vi "Template.vi"() -> ()   [LabVIEW 2021]
uses:
  _Template/_Template/_Template.lvclass
  _Shared/_Shared.lvlib
panel:
  in  "Create":bool
  in  "Template Name":string(combo)
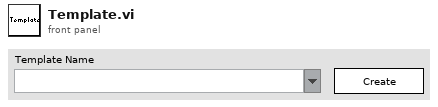
[diagram p1: front panel]
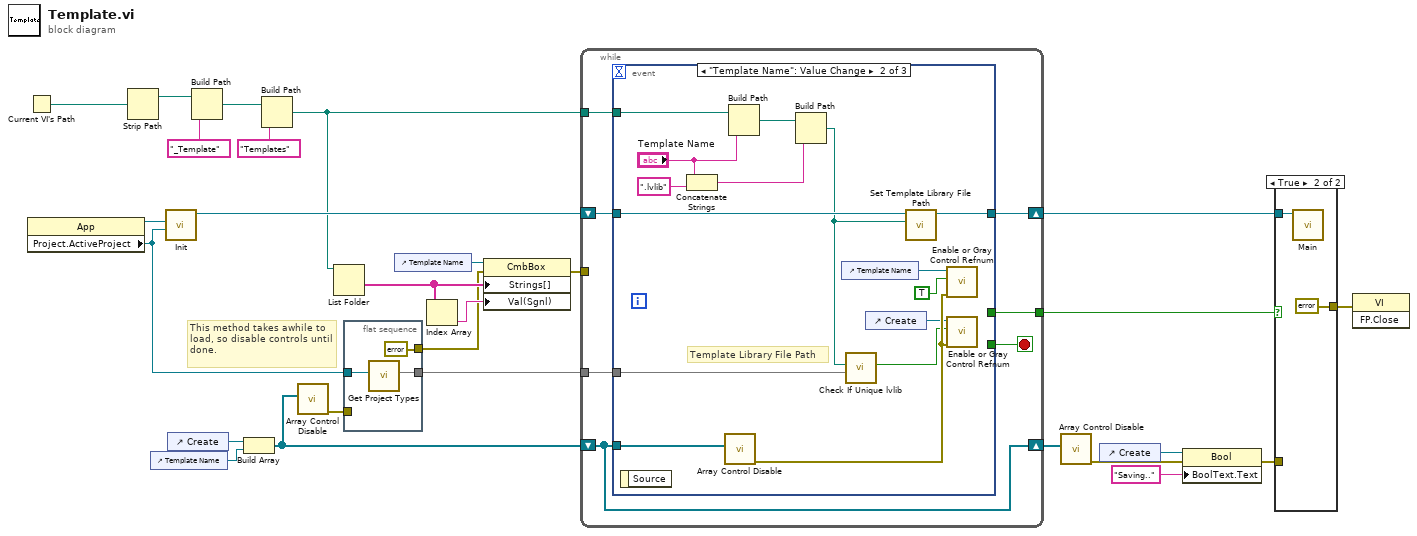
[diagram p0: block diagram]
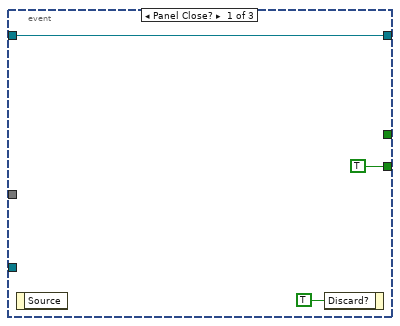
[diagram p2: hidden frame]
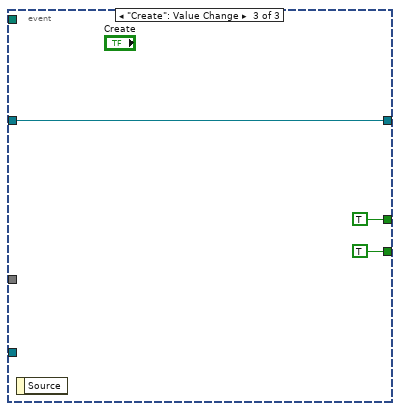
[diagram p3: hidden frame]
diagram:
  # "This method takes awhile to load, so disable controls until done."
  n1 = Current VI's Path() -> (path=w25:path)
  n2 = property class="App"() -> (reference out=w17:refnum<vi>, "Project.ActiveProject"=w14:refnum<vi>)  [unwired: 2 in, 1 out]
  n3 = Strip Path(path=w25) -> (stripped path=w21:path)  [unwired: 1 out]
  n4 = control-ref of="Template Name"() -> (w6:refnum<vi>)
  n5 = call "Init.vi"("Project:Active Project"=w14, "NI.LV.Dialog Instance"=w17) -> ("_Template out"=w18:refnum<class "_Template.lvclass">)  [unwired: 9 in]
  n6 = control-ref of="Create"() -> (w7:refnum<vi>)
  n7 = Build Path(base path=w21, name or relative path="_Template" ("regular expression")) -> (appended path=w22:path)
  n8 = Build Array(w7, w6) -> (w5:refnum<vi>[])
  n9 = Build Path(base path=w22, name or relative path="Templates" ("regular expression")) -> (appended path=w15:path)
  n10 = call "Array Control Disable.vi"("Array Control in"=w5) -> ("error out"=w4:errorcluster)  [unwired: 10 in]
  n11 = List Folder(path=w15) -> (folder names=w11:string[])  [unwired: 3 in, 3 out]
  n12 = flat-sequence {
    tunnel: w14 -> [w30]
    tunnel: [w29] -> w13
    tunnel: [errorcluster {"status"=FALSE, "code"=0, "source"=""} ("error out")] -> w10
    tunnel: w4 -> [_]
    frame #0 {
      n13 = call "Get Project Types.vi"("Project:Active Project"=w30) -> ("Type Name Library File Path"=w29:map{string, map{string, path}})  [unwired: 10 in]
    }
  }
  n14 = control-ref of="Template Name"() -> (w26:refnum<vi>)
  n15 = Index Array(array=w11) -> (element=w12:string)  [unwired: 1 in]
  n16 = property class="CmbBox"(reference=w26, error in=w10, "Strings[]"=w11, "Val(Sgnl)"=w12) -> (error out=w19:errorcluster)  [unwired: 1 out]
  n17 = while {
    tunnel: [w37] -> w27
    tunnel: w19 -> [_]
    shift-right: [w34] -> w16
    shift-left: w18 -> [w35]
    tunnel: w15 -> [w33]
    tunnel: w13 -> [w32]
    shift-right: [w31] -> w3
    shift-left: w5 -> [w31]
    stop <- w36 stop-if-true
    n18 = event shown="[1] \"Template Name\": Value Change" {
      selector: _ -> [_ _ _]
      dyn-events: _ -> [_ _ _]
      timeout: _ -> [_ _ _]
      tunnel: [_ _ TRUE] -> w37
      tunnel: [TRUE ("Discard?") _ TRUE ("Discard?")] -> w36
      tunnel: w35 -> [w38 w48 w56]
      tunnel: [w38 w47 w56] -> w34
      tunnel: w33 -> [_ w53 _]
      tunnel: w32 -> [_ w46 _]
      tunnel: w31 -> [_ w42 _]
      event Panel Close? {
        n19 = event-data() -> ()  [unwired: 1 in, 1 out]
        n20 = event-data("Discard?"=TRUE) -> ()  [unwired: 1 in, 1 out]
      }
      event "Template Name": Value Change {
        # "Template Library File Path"
        n21 = event-data() -> ()  [unwired: 1 in, 1 out]
        n22 = Concatenate Strings("Template Name", ".lvlib" ("string")) -> (w51:string)
        n23 = call "Array Control Disable.vi"("Array Control in"=w42) -> ("error out"=w55:errorcluster)  [unwired: 10 in]
        n24 = Build Path(base path=w53, name or relative path="Template Name") -> (appended path=w52:path)
        n25 = Build Path(base path=w52, name or relative path=w51) -> (appended path=w45:path)
        n26 = control-ref of="Template Name"() -> (w43:refnum<vi>)
        n27 = call "Check If Unique lvlib.vi"("Type Name Library File Path"=w46, "Library File Path"=w45) -> ("Unique?"=w41:bool)  [unwired: 9 in]
        n28 = control-ref of="Create"() -> (w49:refnum<vi>)
        n29 = call "Set Template Library File Path.vi"("Template Library File Path"=w45, "_Template in"=w48) -> ("_Template out"=w47:refnum<class "_Template.lvclass">)  [unwired: 9 in]
        n30 = call <vilib>:"Enable or Gray Control Refnum.vi"("error in (no error)"=w55, "enable?"=TRUE, "Control in"=w43) -> ()  [unwired: 7 in, 2 out]
        n31 = call <vilib>:"Enable or Gray Control Refnum.vi"("error in (no error)"=w55, "enable?"=w41, "Control in"=w49) -> ()  [unwired: 7 in, 2 out]
      }
      event "Create": Value Change {
        n32 = event-data() -> ()  [unwired: 1 in, 1 out]
      }
    }
  }
  n33 = call "Array Control Disable.vi"("Array Control in"=w3) -> ("error out"=w2:errorcluster)  [unwired: 10 in]
  n34 = control-ref of="Create"() -> (w8:refnum<vi>)
  n35 = property class="Bool"(reference=w8, error in=w2, "BoolText.Text"="Saving.." ("Boolean Text.Text")) -> (error out=w9:errorcluster)  [unwired: 1 out]
  n36 = case shown="True" w27 {
    tunnel: [_ errorcluster {"status"=FALSE, "code"=0, "source"=""} ("error in (no error)")] -> w20
    tunnel: w16 -> [_ w59]
    tunnel: w9 -> [_ _]
    frame False {
    }
    frame True {
      n37 = call "Main.vi"("_Template in"=w59) -> ()  [unwired: 11 in]
    }
  }
  n38 = invoke class="VI" method="FP.Close"(error in=w20) -> ()  [unwired: 2 in, 3 out]
